vi "Test Plugins.vi"() -> ()   [LabVIEW 2014]
uses:
  reusable/Sequence/SEQ.lvlibp/STEPS/STEP.lvclass
  Send MSG STEP.lvlibp/Send MSG STEP.lvclass
  <vilib>/Utility/LVLibp/NI_PackedLibraryUtility.lvlib
panel:
  out "specific class reference":refnum<class "STEP.lvclass">
  out "error out":errorcluster
  out "filenames":string[](array[string])
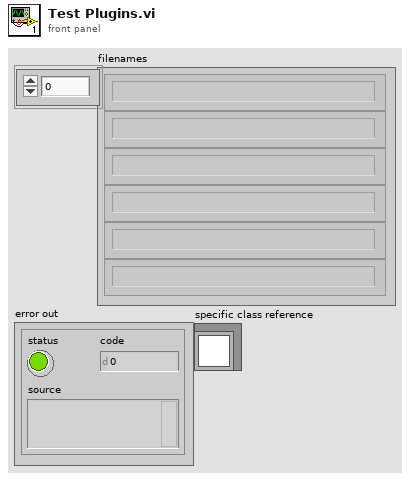
[diagram p1: front panel]
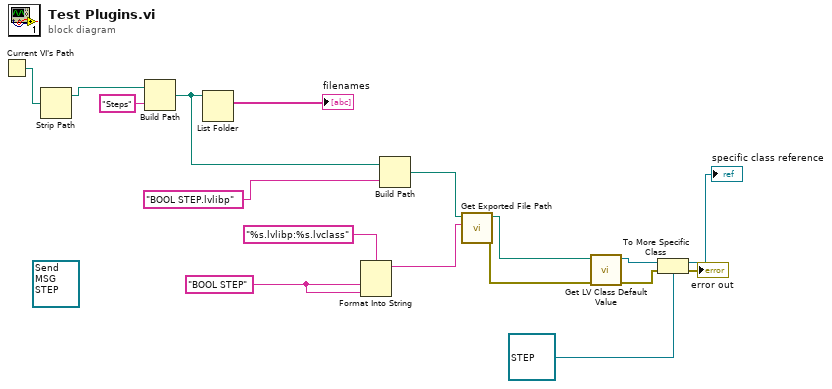
[diagram p0: block diagram]
diagram:
  w9 = "BOOL STEP" ("input 1")
  (unwired) refnum<class "Send MSG STEP.lvclass"> refnum ("Send MSG STEP.lvlibp:Send MSG STEP")
  n1 = Current VI's Path() -> (path=w16:path)
  n2 = Strip Path(path=w16) -> (stripped path=w15:path)  [unwired: 1 out]
  n3 = Build Path(base path=w15, name or relative path="Steps") -> (appended path=w8:path)
  n4 = List Folder(path=w8) -> (filenames=→"filenames":string[])  [unwired: 3 in, 3 out]
  n5 = Format Into String(format string="%s.lvlibp:%s.lvclass", w9, w9) -> (resulting string=w5:string)  [unwired: 2 in, 1 out]
  n6 = Build Path(base path=w8, name or relative path="BOOL STEP.lvlibp" ("input 1")) -> (appended path=w6:path)
  n7 = call <vilib>:"Get Exported File Path.vi"("qualified name"=w5, "packed library path"=w6) -> ("error out"=w3:errorcluster, "path"=w4:path)  [unwired: 8 in]
  n8 = call <vilib>:"Get LV Class Default Value.vi"("error in (no error)"=w3, "class path"=w4) -> ("error out"=w10:errorcluster, "object"=w12:refnum<class>)  [unwired: 8 in]
  n9 = To More Specific Class(target class=refnum<class "STEP.lvclass"> refnum ("Sequence Composition:STEP.lvclass"), reference=w12, error in=w10) -> (specific class reference=→"specific class reference":refnum<class "STEP.lvclass">, error out=→"error out":errorcluster)
